vi "Read stoppedByUser.vi"(8 "error in (no error)":errorcluster, 11 "ExperimentControlEvents in":refnum<class "ExperimentControlEvents.lvclass">) -> (0 "error out":errorcluster, 2 "stoppedByUser":bool, 3 "ExperimentControlEvents out":refnum<class "ExperimentControlEvents.lvclass">)   [LabVIEW 2009, in "Views.lvlib" / "ExperimentControl.lvlib" / "ExperimentControlEvents.lvclass"]
uses:
  ExperimentControlEvents.lvclass
  ExperimentControlEvents.lvclass/ExperimentControlEvents.ctl
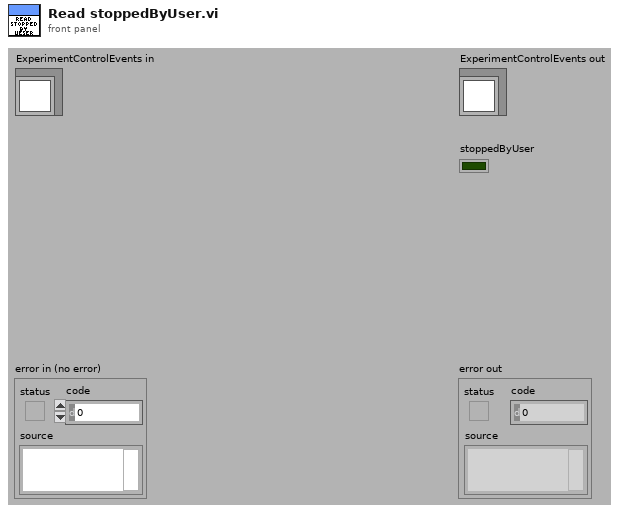
[diagram p1: front panel]
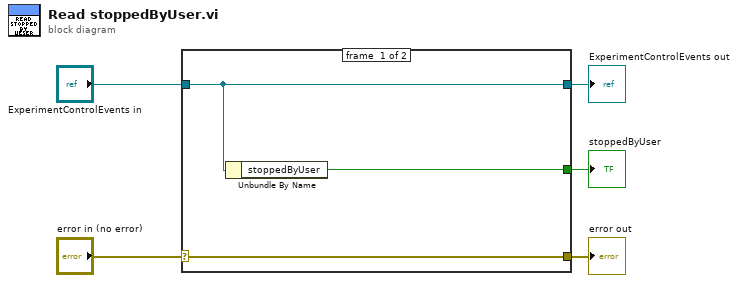
[diagram p0: block diagram]
diagram:
  n1 = case shown="No Error" "error in (no error)" {
    selector: "error in (no error)" -> [w8 w9]
    tunnel: [w8 w9] -> w4
    tunnel: [w7 w10] -> w2
    tunnel: "ExperimentControlEvents in" -> [w7 w10]
    tunnel: [w6 _] -> w1
    frame #0 {
      n2 = Unbundle By Name(w7) -> ("stoppedByUser"=w6:bool)
    }
    frame #1 {
    }
  }
  "error out" <- w4
  "ExperimentControlEvents out" <- w2
  "stoppedByUser" <- w1
